vi "Connect.vi"(8 "error in":errorcluster, 11 "4124 in":refnum<class "4124.lvclass">) -> (0 "error out":errorcluster, 3 "4124 out":refnum<class "4124.lvclass">)   [LabVIEW 2018, in "4124.lvlib" / "4124.lvclass"]
doc: "Connect to NI-4124 Power Supply"
uses:
  4124.lvclass
  <instrlib>/NI RMX-412x Power Supplies/NI RMX-412x Power Supplies.lvlib
  builds/Power_Supply.lvlibp/Power Supply.lvclass
  C:/Users/Ron.Dexter.LUMINARTECH/Desktop/builds/Power_Supply.lvlibp/Power Supply.lvclass
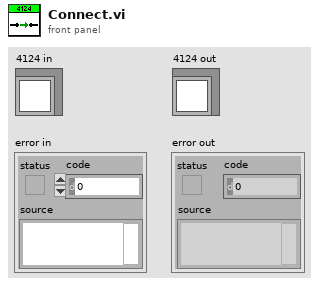
[diagram p1: front panel]
types:
  T1 = cluster{"Baud Rate":u32, "Parity":u16, "Data Bits":u16, "Stop Bits":u16, "Flow Control":u16}
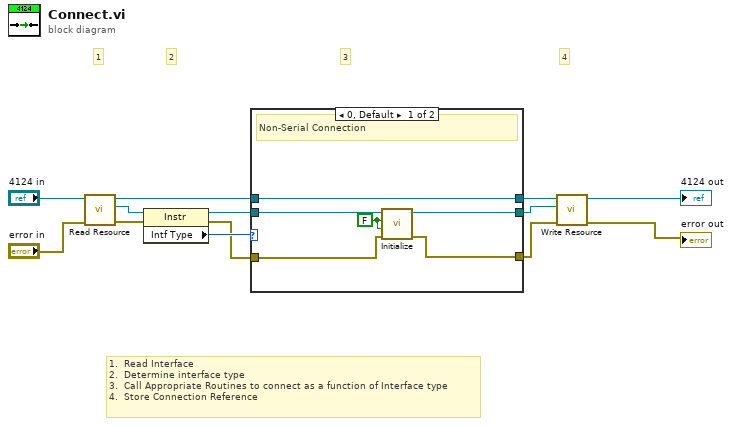
[diagram p0: block diagram]
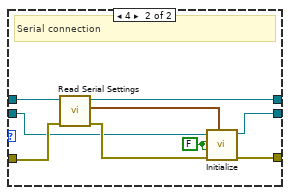
[diagram p2: hidden frame]
diagram:
  # "1.  Read Interface\n2.  Determine interface type\n3.  Call Appropriate Routines to connect as a function of Interface type\n4.  Store Connection Reference"
  # "4"
  # "3"
  # "2"
  # "1"
  n1 = call "Read Resource.vi"("error in"="error in", "Power Supply in"="4124 in") -> ("error out"=w8:errorcluster, "Resource"=w9:refnum<visa-resource-name>, "Power Supply out"=w4:refnum<class "4124.lvclass">)  [unwired: 7 in]
  n2 = property class="Instr"(reference=w9, error in=w8) -> (reference out=w6:refnum<visa-resource-name>, error out=w5:errorcluster, "Intf Type"=w7:u16)
  n3 = case shown="0, Default" w7 {
    tunnel: w6 -> [w17 w20]
    tunnel: w5 -> [w15 w23]
    tunnel: w4 -> [w19 w25]
    tunnel: [w19 w24] -> w3
    tunnel: [w16 w26] -> w2
    tunnel: [w14 w27] -> w1
    frame 0, Default {
      w18 = FALSE ("ID Query (True)")
      # "Non-Serial Connection"
      n4 = call <instrlib>:"Initialize.vi"("error in (no error)"=w15, "Reset (True)"=w18, "ID Query (True)"=w18, "VISA resource name"=w17) -> ("error out"=w14:errorcluster, "VISA resource name out"=w16:refnum<visa-resource-name>)  [unwired: 6 in]
    }
    frame 4 {
      w28 = FALSE ("ID Query (True)")
      # "Serial connection"
      n5 = call "Read Serial Settings.vi"("error in"=w23, "4124 in"=w25) -> ("error out"=w22:errorcluster, "Serial Configuration"=w21:T1, "4124 out"=w24:refnum<class "4124.lvclass">)  [unwired: 7 in]
      n6 = call <instrlib>:"Initialize.vi"("Serial Configuration"=w21, "error in (no error)"=w22, "Reset (True)"=w28, "ID Query (True)"=w28, "VISA resource name"=w20) -> ("error out"=w27:errorcluster, "VISA resource name out"=w26:refnum<visa-resource-name>)  [unwired: 5 in]
    }
  }
  n7 = call "Write Resource.vi"("error in"=w1, "Resource"=w2, "Power Supply in"=w3) -> ("error out"=→"error out":errorcluster, "Power Supply out"=→"4124 out":refnum<class "4124.lvclass">)  [unwired: 7 in]
